vi "scan.vi"(8 "error in (no error)":errorcluster, 11 "Input":string="0,-110n,10n,64") -> (0 "error out":errorcluster, 3 "Output":string)   [LabVIEW 2019]
panel:
  in  "seconds to wait":dbl=3.0
  in  "Angle (deg)":sgl=nan caption="Angle (deg) (NaN=no change)" format="%.2f"
  in  "Size (m)":cluster{"Width":sgl, "Height":sgl}={"Width"=1e-08, "Height"=1e-08} caption="Size (m) (NaN=no change)" {"Height" format="%.2p"; "Width" format="%.2p"}
  out "size(s)":i32=4
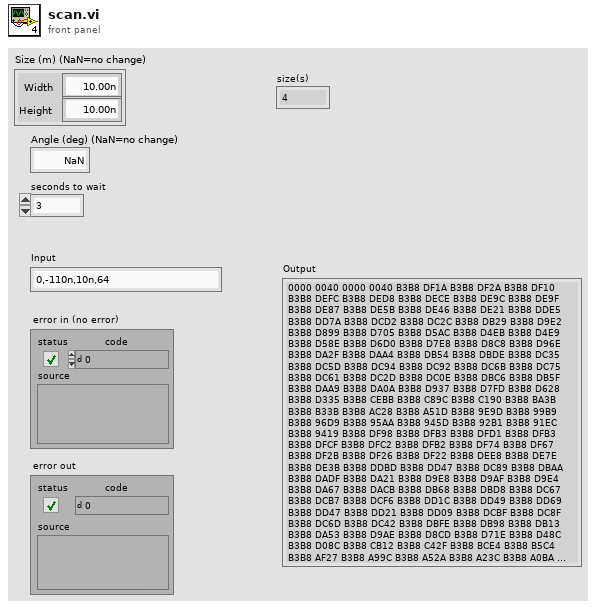
[diagram p1: front panel]
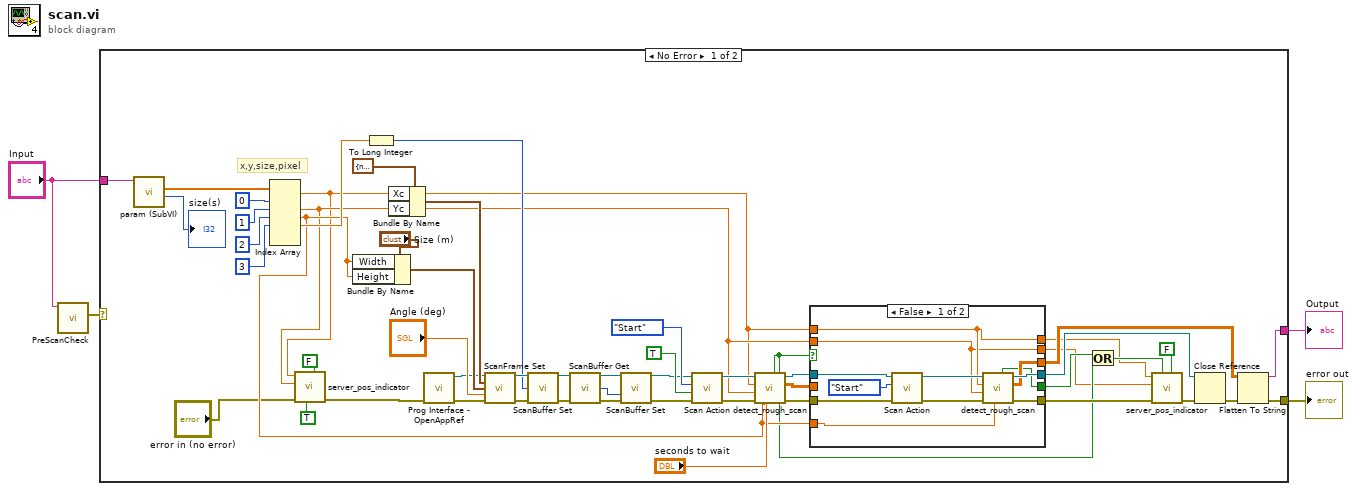
[diagram p0: block diagram]
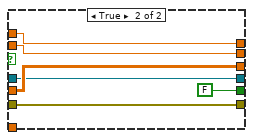
[diagram p2: hidden frame]
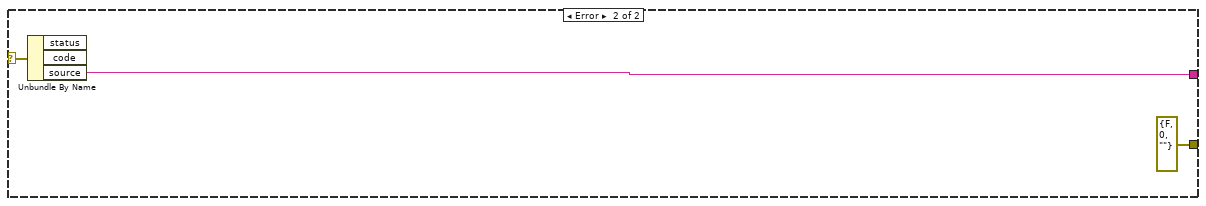
[diagram p3: hidden frame]
diagram:
  n1 = call "PreScanCheck.vi"("Input"="Input") -> ("error"=w1:errorcluster)  [unwired: 8 in, 2 out]
  n2 = case shown="No Error" w1 {
    selector: w1 -> [_ w77]
    tunnel: [w40 w76] -> w4
    tunnel: [w32 errorcluster {"status"=FALSE, "code"=0, "source"=""} ("error out")] -> w3
    tunnel: "Input" -> [w28 _]
    frame No Error {
      # "x,y,size,pixel"
      n3 = call "param (SubVI).vi"("Input"=w28) -> ("num"=→"size(s)":i32, "parm"=w56:dbl[])  [unwired: 8 in, 1 out]
      n4 = Index Array(array=w56, index #1=0 ("index"), index #2=1 ("index"), index #3=2 ("index"), index #4=3 ("index")) -> (element #1=w7:dbl, element #2=w10:dbl, element #3=w20:dbl, element #4=w42:dbl)  [unwired: 2 in, 2 out]
      n5 = call "server_pos_indicator.vi"("reset"=FALSE, "tentative"=TRUE, "error in"="error in (no error)", "yc"=w10, "xc"=w7) -> ("error out"=w11:errorcluster)  [unwired: 6 in]
      n6 = Bundle By Name(cluster="Size (m)", "Width"=w20, "Height"=w20) -> (w43:cluster{"Width":sgl, "Height":sgl})
      n7 = To Long Integer(number=w42) -> (32bit integer=w41:i32)
      n8 = Bundle By Name(cluster=cluster{"Xc":sgl, "Yc":sgl} {"Xc"=nan, "Yc"=nan} ("Center coordinates (m)"), "Xc"=w7, "Yc"=w10) -> (w54:cluster{"Xc":sgl, "Yc":sgl})
      n9 = call <userlib>:"Prog Interface - OpenAppRef.vi"("Error in (no error)"=w11) -> ("Error out"=w19:errorcluster, "Application reference"=w29:refnum<vi>)  [unwired: 5 in]
      n10 = call <userlib>:"ScanFrame Set.vi"("Application ref in"=w29, "Center coordinates (m)"=w54, "Size (m)"=w43, "Angle (deg)"="Angle (deg)", "error in (no error)"=w19) -> ("Application ref out"=w52:refnum<vi>, "error out"=w51:errorcluster)  [unwired: 9 in]
      n11 = call <userlib>:"ScanBuffer Set.vi"("Application ref in"=w52, "Pixels"=w41, "error in (no error)"=w51) -> ("Application ref out"=w36:refnum<vi>, "error out"=w35:errorcluster)  [unwired: 11 in]
      n12 = call <userlib>:"ScanBuffer Get.vi"("Application ref in"=w36, "error in (no error)"=w35) -> ("Application ref out"=w38:refnum<vi>, "Pixels/line"=w39:i32, "error out"=w37:errorcluster)  [unwired: 9 in, 2 out]
      n13 = call <userlib>:"ScanBuffer Set.vi"("Application ref in"=w38, "Lines"=w39, "error in (no error)"=w37) -> ("Application ref out"=w34:refnum<vi>, "error out"=w33:errorcluster)  [unwired: 11 in]
      n14 = call <userlib>:"Scan Action.vi"("error in (no error)"=w33, "Direction: up/down (T=up)"=TRUE, "Scan action (Start)"=enum16{"Start", "Stop", "Pause", "Resume"}."Start", "Application ref in"=w34) -> ("error out"=w23:errorcluster, "Application ref out"=w24:refnum<vi>)  [unwired: 5 in]
      n15 = call "detect_rough_scan.vi"("size (m)"=w20, "max scan time"="seconds to wait", "Error in"=w23, "Y (m)"=w10, "X (m)"=w7, "App in"=w24) -> ("error out"=w18:errorcluster, "Array"=w21:sgl[][], "Application ref out"=w22:refnum<vi>, "rough image detected"=w14:bool)  [unwired: 2 in]
      n16 = case shown="False" w14 {
        tunnel: [w69 w74] -> w27
        tunnel: [w68 w73] -> w17
        tunnel: [w66 w75] -> w26
        tunnel: w22 -> [w64 w74]
        tunnel: w18 -> [w63 w73]
        tunnel: w21 -> [_ w75]
        tunnel: w7 -> [w60 w71]
        tunnel: w10 -> [w59 w70]
        tunnel: w20 -> [w62 _]
        tunnel: [w61 FALSE ("rough image detected")] -> w13
        tunnel: [w60 w71] -> w6
        tunnel: [w59 w70] -> w5
        frame False {
          n17 = call <userlib>:"Scan Action.vi"("error in (no error)"=w63, "Scan action (Start)"=enum16{"Start", "Stop", "Pause", "Resume"}."Start", "Application ref in"=w64) -> ("error out"=w58:errorcluster, "Application ref out"=w67:refnum<vi>)  [unwired: 6 in]
          n18 = call "detect_rough_scan.vi"("size (m)"=w62, "Error in"=w58, "Y (m)"=w59, "X (m)"=w60, "App in"=w67) -> ("error out"=w68:errorcluster, "Array"=w66:sgl[][], "Application ref out"=w69:refnum<vi>, "rough image detected"=w61:bool)  [unwired: 3 in]
        }
        frame True {
        }
      }
      n19 = Or(x=w13, y=w14) -> (x .or. y?=w15:bool)
      n20 = call "server_pos_indicator.vi"("reset"=FALSE, "rough"=w15, "error in"=w17, "yc"=w5, "xc"=w6) -> ("error out"=w16:errorcluster)  [unwired: 6 in]
      n21 = Close Reference(reference=w27, error in (no error)=w16) -> (error out=w30:errorcluster)
      n22 = Flatten To String(anything=w26, error in (no error)=w30) -> (data string=w40:string, error out=w32:errorcluster)  [unwired: 2 in, 1 out]
    }
    frame Error {
      n23 = Unbundle By Name(w77) -> ("source"=w76:string)  [unwired: 2 out]
    }
  }
  "Output" <- w4
  "error out" <- w3
